vi "Framework.Get Debug Flags.vi"(11 "Framework in":refnum<class "Framework.lvclass">) -> (2 "Debug Flags":refnum<class "Debug Flags.lvclass">, 3 "Framework out":refnum<class "Framework.lvclass">)   [LabVIEW 2017, in "DSF Core.lvlib" / "Framework.lvclass"]
uses:
  Framework.lvclass
  Debug/Debug Flags.lvclass
  Framework.lvclass/Framework.ctl
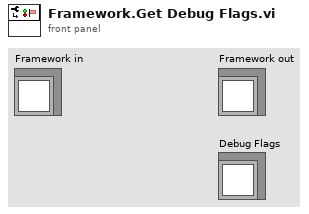
[diagram p1: front panel]
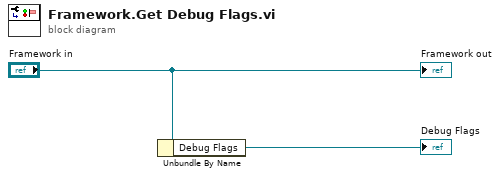
[diagram p0: block diagram]
diagram:
  n1 = Unbundle By Name("Framework in") -> ("Debug Flags"=→"Debug Flags":refnum<class "Debug Flags.lvclass">)
  "Framework out" <- "Framework in"
